vi "LED_top_interp.vi"(5 "FPGA I/O In":refnum<k21>="IO Module\\D0 0", 7 "Testpulser On/Off":bool, 8 "State In":enum16{"Initialize", "Get New Value", "Wait"}(ring), 9 "Testpulse Time Delay (20 ns ticks)":u32=15, 10 "Testpulse duration (20 ns ticks)":u32=1, 11 "Address In":u16) -> (0 "Is Test Pulse?":bool)   [LabVIEW 2012]
uses:
  <vilib>/rvi/FXPMathLib/FxpMul/XNode/nifxpmath_Multiplier.xnode
  <vilib>/rvi/FXPMathLib/sim/FxpSim.dll
panel:
  out "Randomly generated testpulse separation input (20 ns ticks)":u32=50000
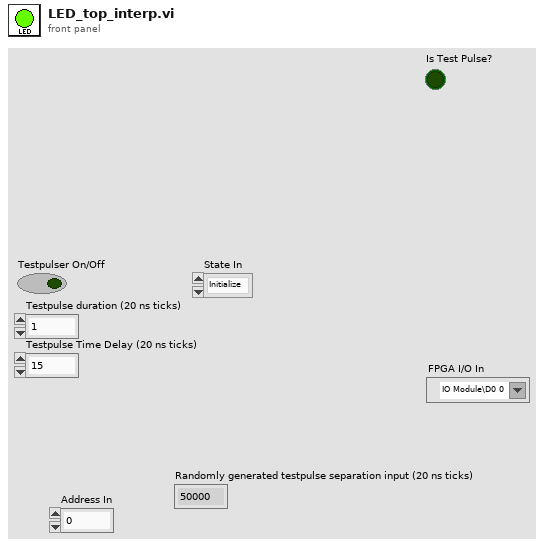
[diagram p1: front panel]
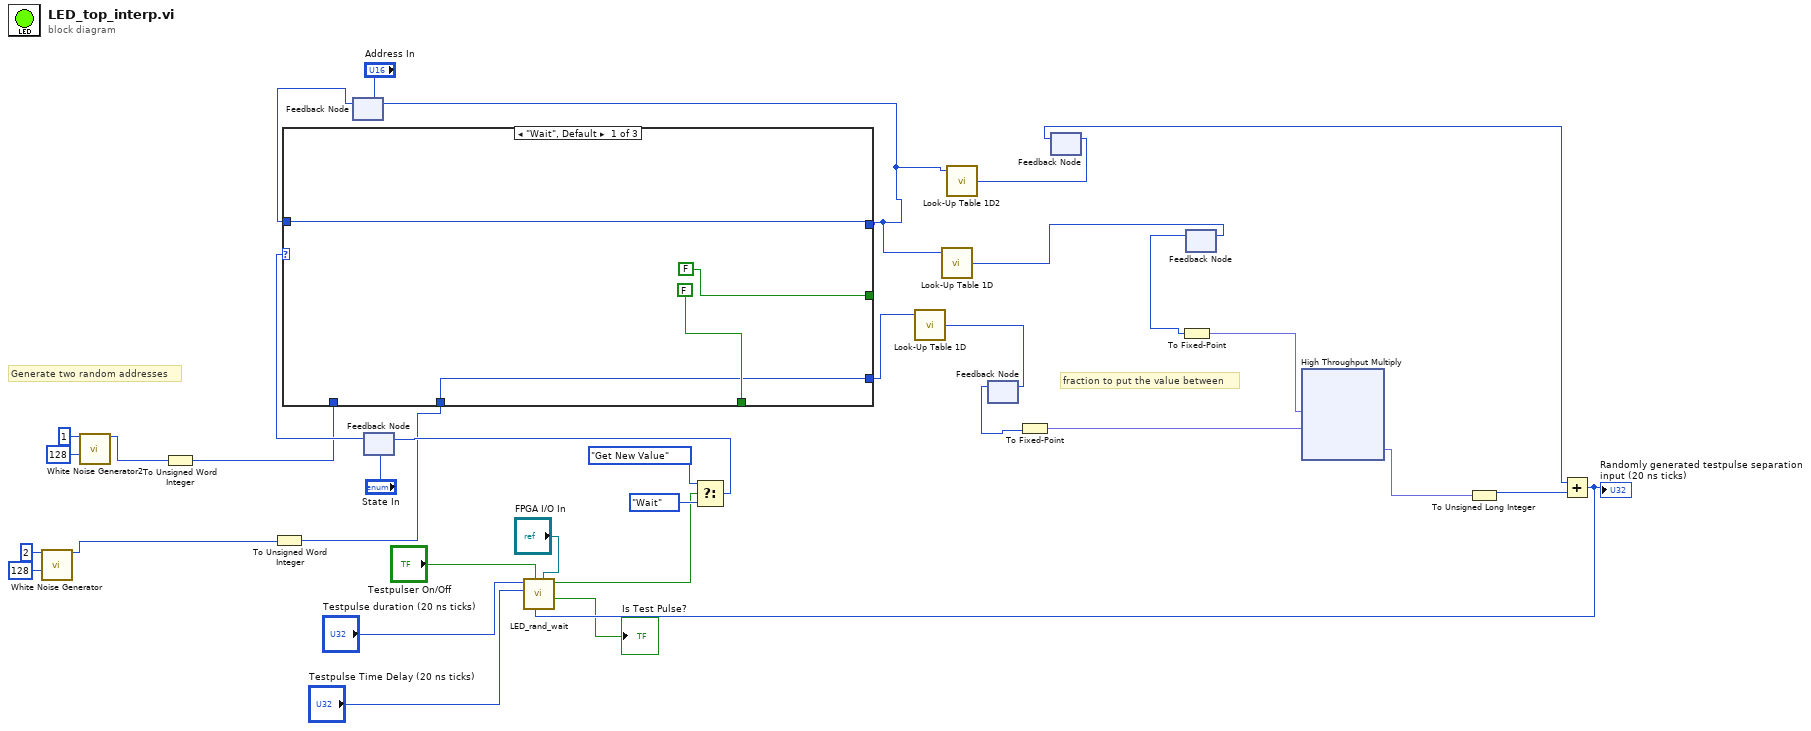
[diagram p0: block diagram]
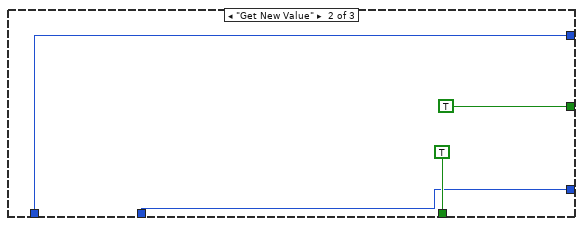
[diagram p2: hidden frame]
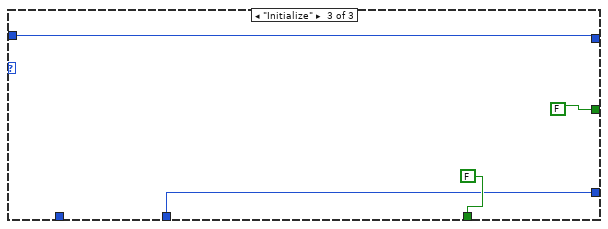
[diagram p3: hidden frame]
diagram:
  # "Generate two random addresses"
  # "fraction to put the value between"
  n1 = call "White Noise Generator"("seed"=u32 2, "amplitude"=u16 128) -> ("white noise out"=w4:i16)  [unwired: 13 in]
  n2 = call "White Noise Generator2"("seed"=u32 1, "amplitude"=u16 128) -> ("white noise out"=w3:i16)  [unwired: 13 in]
  n3 = To Unsigned Word Integer(number=w3) -> (unsigned 16bit integer=w2:u16)
  n4 = To Unsigned Word Integer(number=w4) -> (unsigned 16bit integer=w16:u16)
  n5 = feedback #1("Address In") -> (w24:u16)
  n6 = feedback #2("State In") -> (w30:enum16{"Initialize", "Get New Value", "Wait"})
  n7 = case shown="\"Wait\", Default" w30 {
    tunnel: w24 -> [w36 _ w44]
    tunnel: [FALSE TRUE FALSE] -> _
    tunnel: [FALSE TRUE FALSE] -> _
    tunnel: [w35 w40 w43] -> w15
    tunnel: w16 -> [w35 w40 w43]
    tunnel: w2 -> [_ w39 _]
    tunnel: [w36 w39 w44] -> w7
    frame "Wait", Default {
    }
    frame "Get New Value" {
    }
    frame "Initialize" {
    }
  }
  n8 = feedback-in #1(w7) -> ()
  n9 = call "Look-Up Table 1D"("address"=w15) -> ("data out"=w22:u16)  [unwired: 8 in]
  n10 = call "Look-Up Table 1D"("address"=w7) -> ("data out"=w20:u32)  [unwired: 8 in]
  n11 = call "Look-Up Table 1D2"("address"=w7) -> ("data out"=w6:u32)  [unwired: 8 in]
  n12 = feedback #3() -> (w19:u16)  [unwired: 1 in]
  n13 = feedback-in #3(w22) -> ()
  n14 = To Fixed-Point(number=w19) -> (fixed-point=w8:fxp<+,5,0>)  [unwired: 1 in]
  n15 = feedback #4() -> (w5:u32)  [unwired: 1 in]
  n16 = feedback-in #4(w6) -> ()
  n17 = feedback #5() -> (w9:u32)  [unwired: 1 in]
  n18 = To Fixed-Point(number=w9) -> (fixed-point=w11:fxp<+,15,15>)  [unwired: 1 in]
  n19 = feedback-in #5(w20) -> ()
  n20 = xnode ("High Throughput Multiply")("x"=w11, "y"=w8) -> ("x*y"=w10:fxp<+,15,15>)
  n21 = To Unsigned Long Integer(number=w10) -> (unsigned 32bit integer=w21:u32)
  n22 = Add(x=w5, y=w21) -> (x+y=w23:u32)
  "Randomly generated testpulse separation input (20 ns ticks)" <- w23
  n23 = call "LED_rand_wait.vi"("FPGA I/O In"="FPGA I/O In", "Randomly generated testpulse separation input (20 ns ticks)"=w23, "Testpulser On/Off"="Testpulser On/Off", "Testpulse Time Delay (20 ns ticks)"="Testpulse Time Delay (20 ns ticks)", "Testpulse duration (20 ns ticks)"="Testpulse duration (20 ns ticks)") -> ("Is Test Pulse?"=→"Is Test Pulse?":bool, "Get New Value"=w14:bool)  [unwired: 5 in]
  n24 = Select(t=enum16{"Initialize", "Get New Value", "Wait"}."Get New Value", s=w14, f=enum16{"Initialize", "Get New Value", "Wait"}."Wait") -> (s? t:f=w32:enum16{"Initialize", "Get New Value", "Wait"})
  n25 = feedback-in #2(w32) -> ()
